vi "Calibration Cal Execute Set Cal Executed.vi"(8 "error in (no error)":errorcluster, 10 "Cal Executed":bool, 11 "niDTS Calibration Cal Execute RF Test in":refnum<class "niDTS Calibration Cal Execute RF Test.lvclass">) -> (0 "error out":errorcluster, 3 "niDTS Calibration Cal Execute RF Test out":refnum<class "niDTS Calibration Cal Execute RF Test.lvclass">)   [LabVIEW 2015, in "niDTS Utilities.lvlib" / "niDTS Calibration Cal Execute RF Test.lvclass"]
uses:
  niDTS Calibration Cal Execute RF Test.lvclass
  niDTS Calibration Cal Execute RF Test.lvclass/niDTS Calibration Cal Execute RF Test.ctl
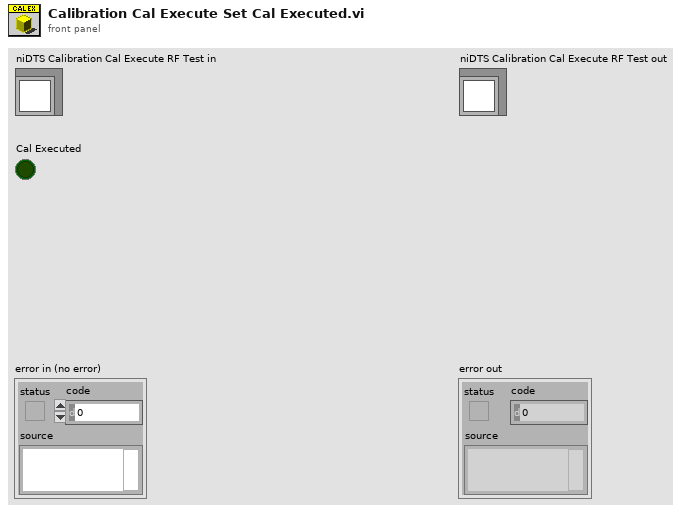
[diagram p1: front panel]
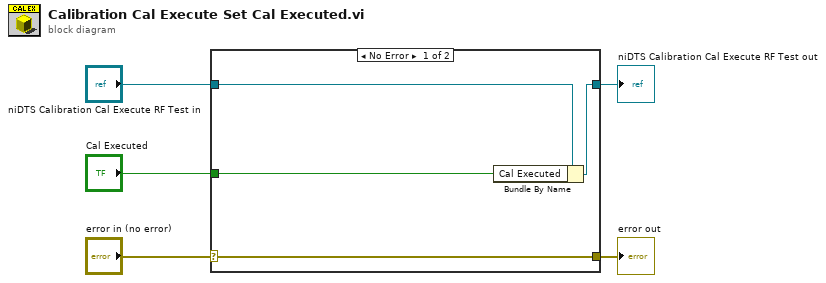
[diagram p0: block diagram]
diagram:
  n1 = case shown="No Error" "error in (no error)" {
    selector: "error in (no error)" -> [w9 w10]
    tunnel: [w9 w10] -> w4
    tunnel: [w7 w11] -> w2
    tunnel: "niDTS Calibration Cal Execute RF Test in" -> [w8 w11]
    tunnel: "Cal Executed" -> [w6 _]
    frame No Error {
      n2 = Bundle By Name(cluster=w8, "Cal Executed"=w6) -> (w7:refnum<class "niDTS Calibration Cal Execute RF Test.lvclass">)
    }
    frame Error {
    }
  }
  "error out" <- w4
  "niDTS Calibration Cal Execute RF Test out" <- w2
